vi "Decode32bitRead.vi"(10 "Read":string="This is simulation mode") -> (2 "Value":i32)   [LabVIEW 2018]
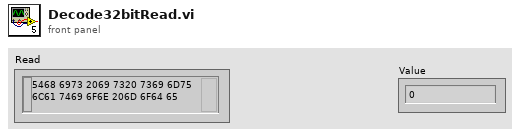
[diagram p1: front panel]
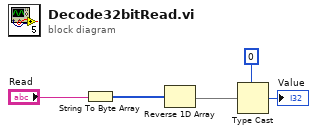
[diagram p0: block diagram]
diagram:
  n1 = String To Byte Array(string="Read") -> (unsigned byte array=w4:u8[])
  n2 = Reverse 1D Array(array=w4) -> (reversed array=w3:u8[])
  n3 = Type Cast(type=0, x=w3) -> (*(type *) &x=→"Value":i32)
